vi "test - Get Filter String - 1.vi"(8 "error in (no error)":errorcluster, 11 "TestCase in":refnum<class "String Filter Tester.lvclass">) -> (0 "error out":errorcluster, 3 "TestCase out":refnum<class "String Filter Tester.lvclass">)   [LabVIEW 2017, in "String Filter Tester.lvclass"]
uses:
  String Filter Tester.lvclass
  Core/Assert API Components/Filter Configurations/String Filters/String Filters.lvclass
  <vilib>/addons/_JKI Toolkits/VI Tester/TestCase.llb/TestCase.lvclass
  C:/Program Files (x86)/National Instruments/LabVIEW 2017/vi.lib/addons/_JKI Toolkits/VI Tester/TestCase.llb/TestCase.lvclass
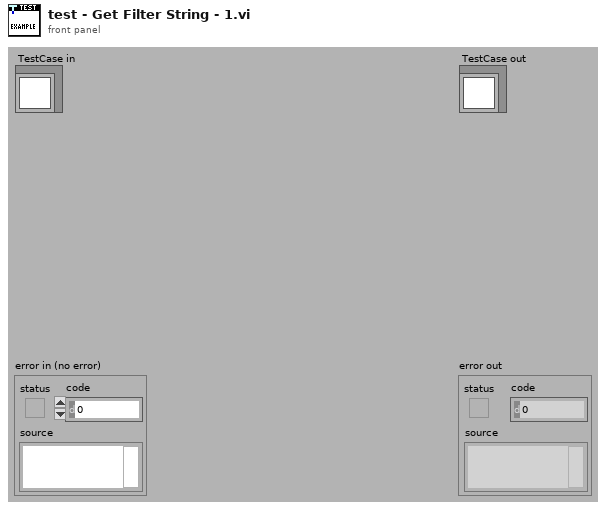
[diagram p1: front panel]
types:
  T1 = enum16{"Contains", "Does Not Contain", "Starts With", "Equals", "Does Not Equal"}
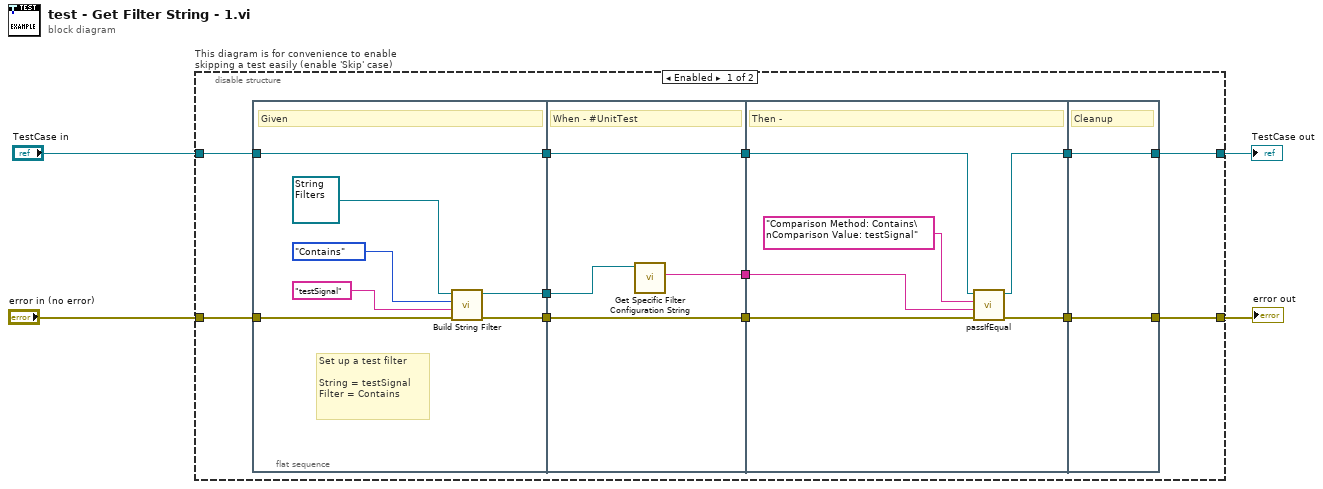
[diagram p0: block diagram]
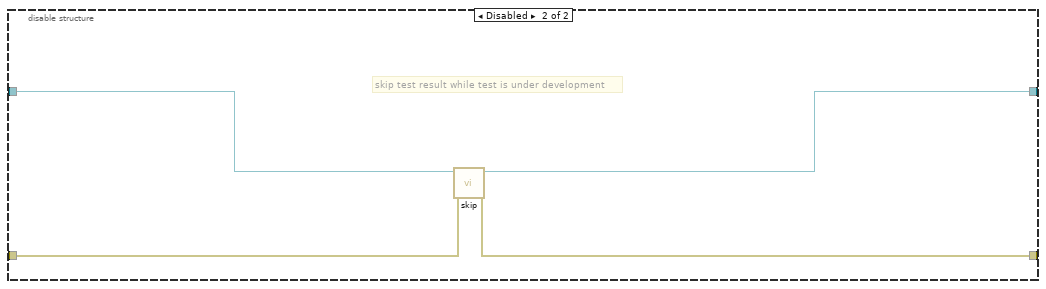
[diagram p2: hidden frame]
diagram:
  n1 = disable-structure "This diagram is for convenience to enable skipping a test easily (enable 'Skip' case)" shown="Enabled" {
    disable-tunnel: "TestCase in" -> [w10 w39]
    disable-tunnel: [w7 w37] -> w1
    disable-tunnel: [w8 w38] -> w3
    disable-tunnel: "error in (no error)" -> [w9 w36]
    frame Enabled {
      n2 = flat-sequence {
        tunnel: w9 -> [w22]
        tunnel: w10 -> [w23]
        tunnel: [w23] -> w16
        tunnel: [w21] -> w15
        tunnel: [w17] -> w6
        tunnel: [w27] -> w14
        tunnel: [w24] -> w13
        tunnel: w16 -> [w27]
        tunnel: w15 -> [w24]
        tunnel: w6 -> [w26]
        tunnel: [w25] -> w5
        tunnel: [w32] -> w12
        tunnel: [w30] -> w11
        tunnel: w14 -> [w33]
        tunnel: w13 -> [w31]
        tunnel: w5 -> [w29]
        tunnel: [w34] -> w8
        tunnel: [w35] -> w7
        tunnel: w12 -> [w35]
        tunnel: w11 -> [w34]
        frame #0 {
          # "Set up a test filter\n\nString = testSignal \nFilter = Contains"
          # "Given"
          n3 = call-dynamic "Build String Filter.vi"("error in (no error)"=w22, "Comparison Value"="testSignal", "Comparison Method"=T1."Contains", "String Filters in"=refnum<class "String Filters.lvclass"> refnum) -> ("error out"=w21:errorcluster, "String Filters out"=w17:refnum<class "String Filters.lvclass">)  [unwired: 6 in]
        }
        frame #1 {
          # "When - #UnitTest"
          n4 = call-dynamic "Get Specific Filter Configuration String.vi"("String Filters in"=w26) -> ("Filter String"=w25:string)  [unwired: 10 in]
        }
        frame #2 {
          # "Then -"
          n5 = call-dynamic "passIfEqual.vi"("error in (no error)"=w31, "y"=w29, "x"="Comparison Method: Contains\nComparison Value: testSignal", "TestCase in"=w33) -> ("error out"=w30:errorcluster, "TestCase out"=w32:refnum<class "String Filter Tester.lvclass">)  [unwired: 6 in]
        }
        frame #3 {
          # "Cleanup"
        }
      }
    }
    frame Disabled {
      # "skip test result while test is under development"
      n6 = call <vilib>:"skip.vi"("error in (no error)"=w36, "TestCase in"=w39) -> ("error out"=w38:errorcluster, "TestCase out"=w37:refnum<class "String Filter Tester.lvclass">)  [unwired: 8 in]
    }
  }
  "error out" <- w3
  "TestCase out" <- w1
